vi "DRAFT2.vi"() -> ()   [LabVIEW 2021]
uses:
  <vilib>/Analysis/3filter.llb/Butterworth Filter (DBL).vi
  <vilib>/Analysis/NI_AALBase.lvlib
  <vilib>/ptbypt/NI_PtbyPt.lvlib
panel:
  out "Array Size 2":u32
  out "Array Size":u32
  out "Elapsed time in ms":u32
  in  "stop":bool
  in  "error in (no error)":errorcluster
  out "error out":errorcluster
  in  "loop 1":i32
  out "Waveform Graph 6":dynamicdata(graph)
  out "Waveform Graph 5":dynamicdata(graph)
  out "Waveform Graph 4":dynamicdata(graph)
  out "Waveform Graph 3":dbl[](graph)
  out "Waveform Graph 2":dynamicdata(graph)
  in  "Boolean":bool
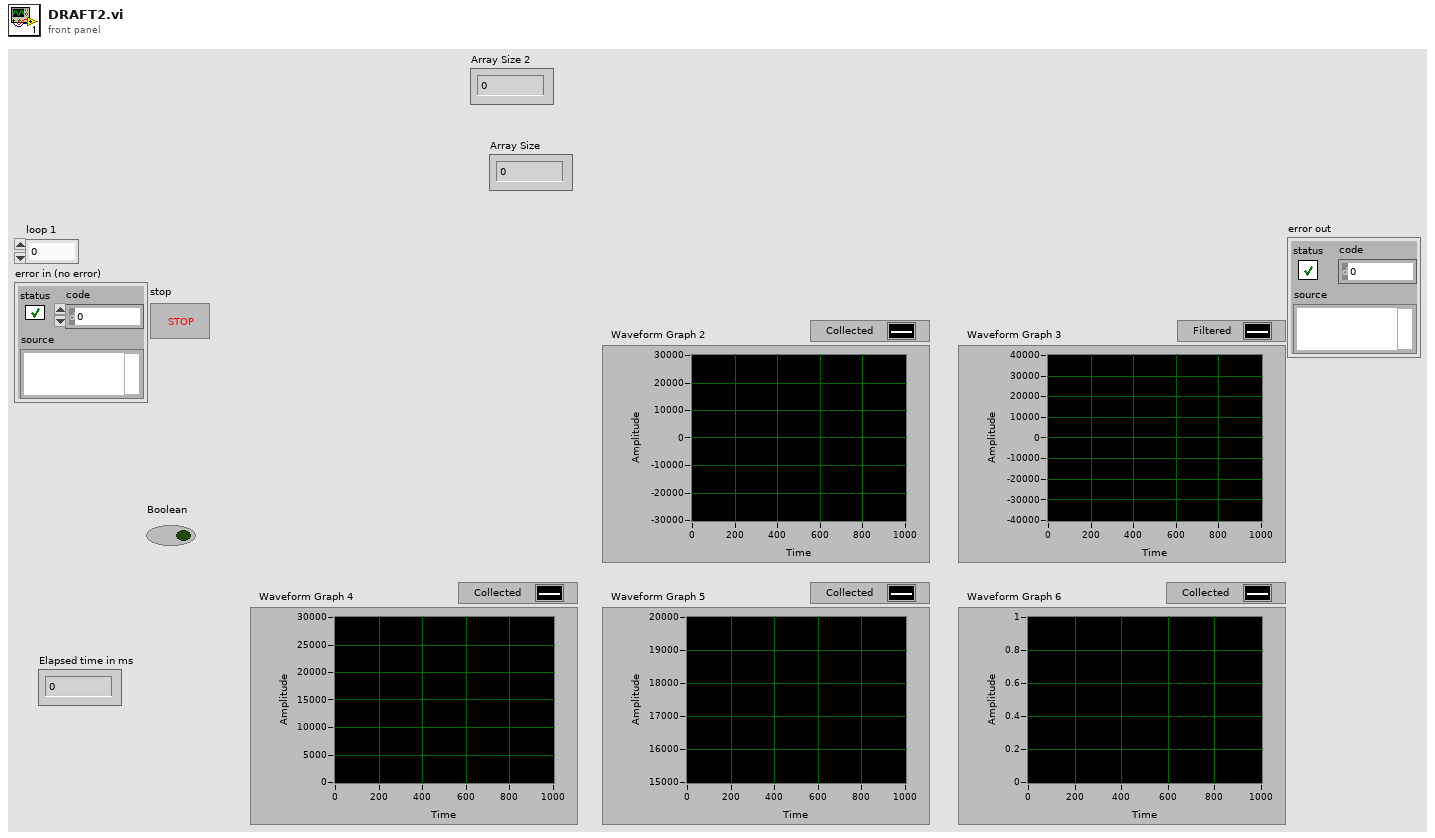
[diagram p1: front panel]
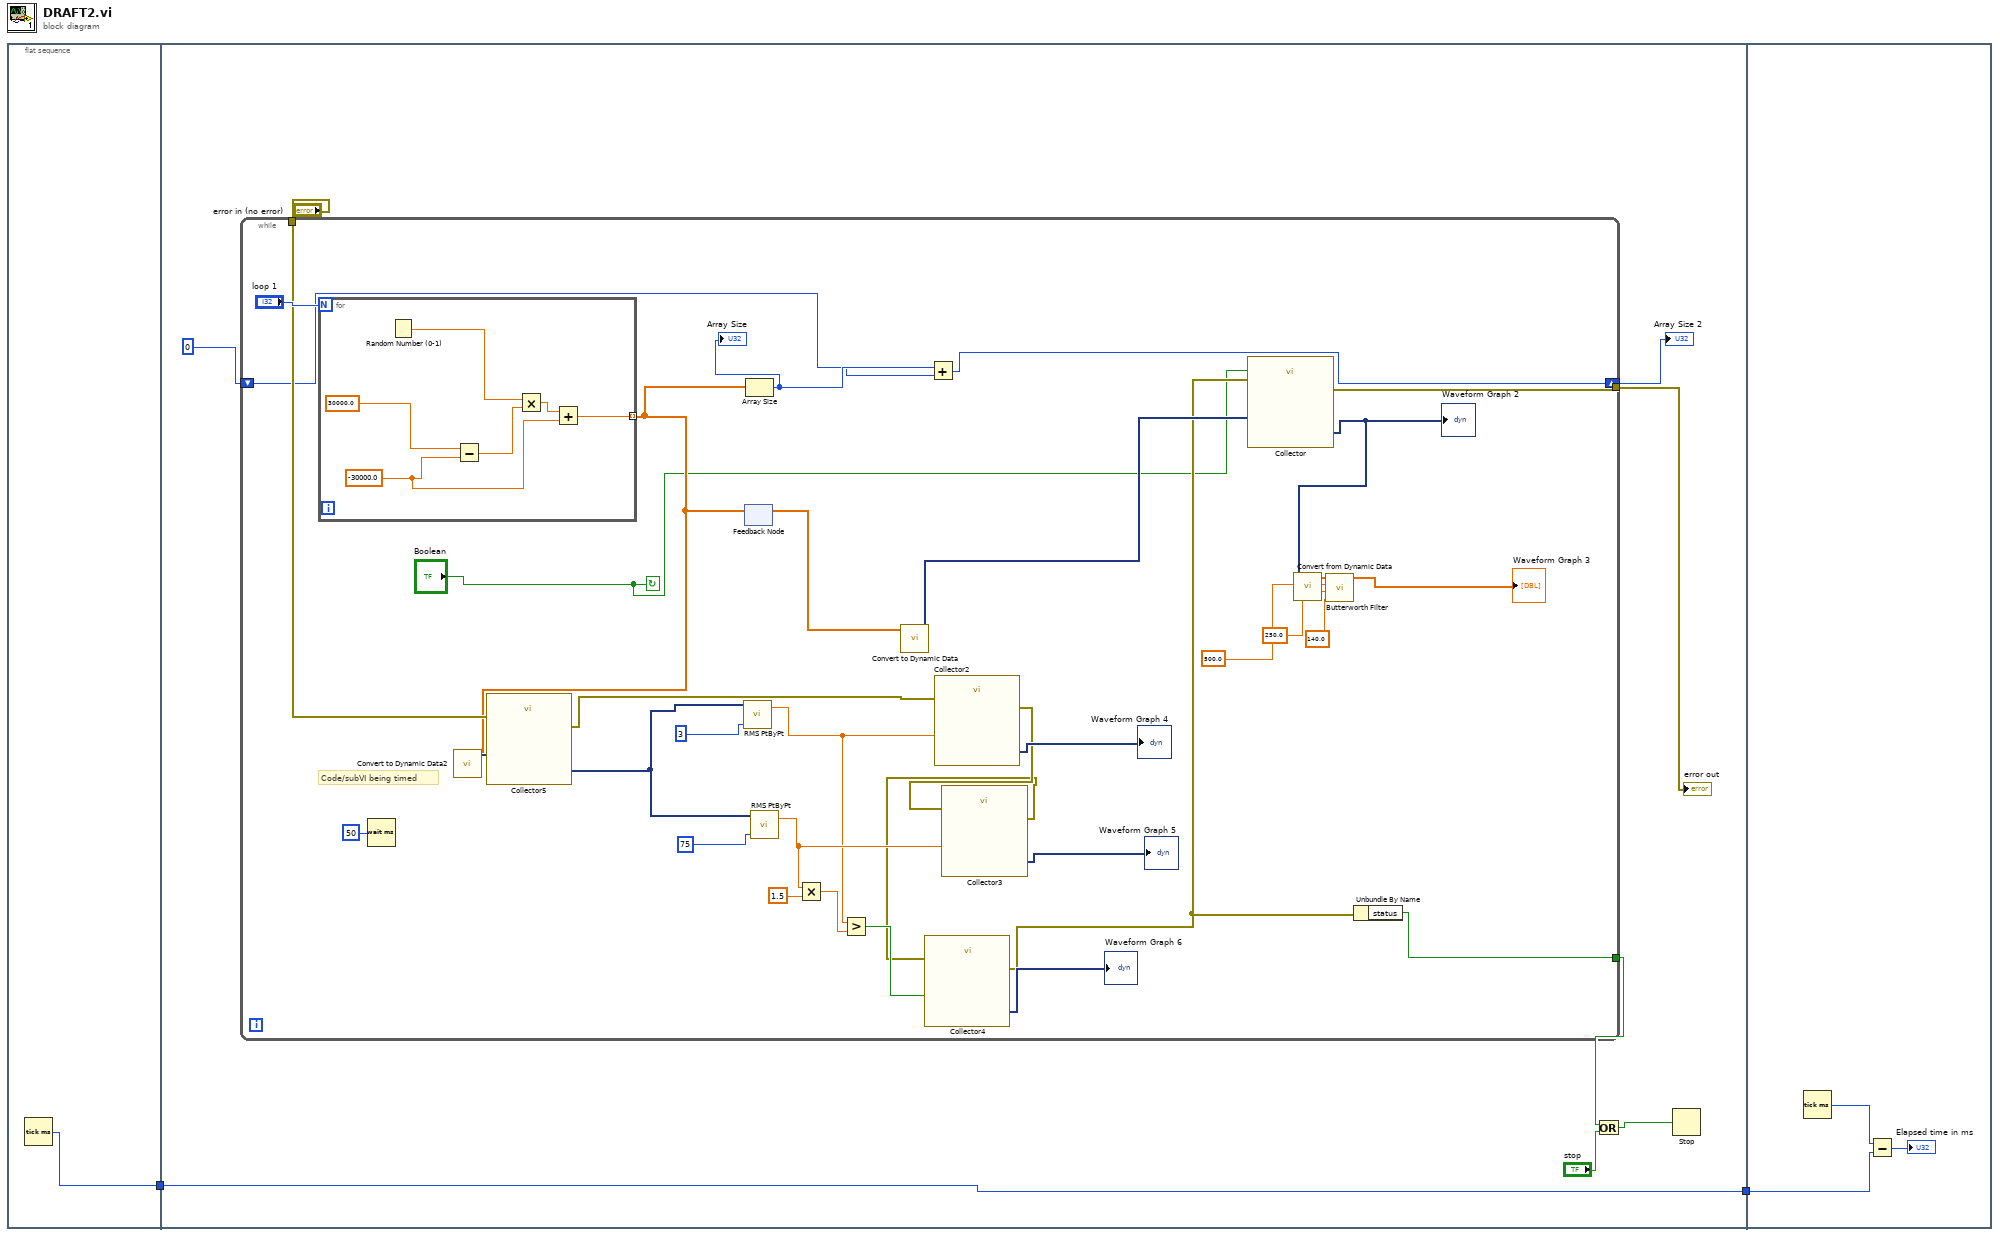
[diagram p0: block diagram]
diagram:
  n1 = flat-sequence {
    tunnel: [w3] -> w2
    tunnel: [w12] -> w1
    tunnel: w2 -> [w12]
    tunnel: w1 -> [w52]
    frame #0 {
      n2 = Tick Count (ms)() -> (millisecond timer value=w3:u32)
    }
    frame #1 {
      # "Code/subVI being timed"
      n3 = while {
        tunnel: "error in (no error)" -> [w25]
        tunnel: [w21] -> w9
        tunnel: [w19] -> w8
        shift-right: [w13] -> w4
        shift-left: 0 -> [w14]
        stop <- "Boolean" continue-if-true
        n4 = for {
          N: "loop 1" -> [_]
          tunnel: [w46] -> w17 mode=indexing
          w48 = -30000.0 ("y")
          n5 = Random Number (0-1)() -> (number: 0 to 1=w47:dbl)
          n6 = Subtract(x=30000.0, y=w48) -> (x-y=w51:dbl)
          n7 = Multiply(x=w47, y=w51) -> (x*y=w50:dbl)
          n8 = Add(x=w50, y=w48) -> (x+y=w46:dbl)
        }
        n9 = call "Convert to Dynamic Data2"("Array"=w17) -> ("Dynamic Data Type"=w27:dynamicdata)  [unwired: 3 in]
        n10 = call "Collector5"("error in (no error)"=w25, "Signals"=w27) -> ("error out"=w24:errorcluster, "Collected Signals"=w26:dynamicdata)  [unwired: 8 in]
        n11 = call <vilib>:"RMS PtByPt.vi"("sample length"=3, "x"=w26) -> ("rms value"=w31:dbl)  [unwired: 2 in, 1 out]
        n12 = feedback-in #1(w17) -> ()
        n13 = feedback #1() -> (w18:dbl[])  [unwired: 1 in]
        n14 = Array Size(array=w17) -> (size(s)=w16:i32)
        "Array Size" <- w16
        n15 = call <vilib>:"RMS PtByPt.vi"("sample length"=75, "x"=w26) -> ("rms value"=w34:dbl)  [unwired: 2 in, 1 out]
        n16 = Multiply(x=w34, y=1.5) -> (x*y=w32:dbl)
        n17 = Greater?(x=w31, y=w32) -> (0:w30:bool)
        n18 = call "Convert to Dynamic Data"("Array"=w18) -> ("Dynamic Data Type"=w37:dynamicdata)  [unwired: 3 in]
        n19 = Add(x=w16, y=w14) -> (x+y=w13:i32)
        n20 = call "Collector2"("error in (no error)"=w24, "Signals"=w31) -> ("error out"=w23:errorcluster, "Collected Signals"=→"Waveform Graph 4":dynamicdata)  [unwired: 8 in]
        n21 = call "Collector3"("error in (no error)"=w23, "Signals"=w34) -> ("error out"=w22:errorcluster, "Collected Signals"=→"Waveform Graph 5":dynamicdata)  [unwired: 8 in]
        n22 = call "Collector4"("error in (no error)"=w22, "Signals"=w30) -> ("error out"=w20:errorcluster, "Collected Signals"=→"Waveform Graph 6":dynamicdata)  [unwired: 8 in]
        n23 = call "Collector"("error in (no error)"=w20, "Enable"="Boolean", "Signals"=w37) -> ("error out"=w21:errorcluster, "Collected Signals"=w40:dynamicdata)  [unwired: 7 in]
        "Waveform Graph 2" <- w40
        n24 = call "Convert from Dynamic Data"("Dynamic Data Type"=w40) -> ("Array"=w42:dbl[])  [unwired: 3 in]
        n25 = call-poly <vilib>:"Butterworth Filter.vi"("low cutoff freq: fl"=140.0, "high cutoff freq: fh"=250.0, "sampling freq: fs"=500.0, "X"=w42) -> ("Filtered X"=→"Waveform Graph 3":dbl[])  [unwired: 4 in, 1 out]
        n26 = Unbundle By Name(w20) -> ("status"=w19:bool)
      }
      "error out" <- w9
      "Array Size 2" <- w4
      n27 = Wait (ms)(milliseconds to wait=u32 50) -> ()  [unwired: 1 out]
      n28 = Or(x=w8, y="stop") -> (x .or. y?=w6:bool)
      n29 = Stop(stop? (T)=w6) -> ()
    }
    frame #2 {
      n30 = Tick Count (ms)() -> (millisecond timer value=w54:u32)
      n31 = Subtract(x=w54, y=w52) -> (x-y=→"Elapsed time in ms":u32)
    }
  }
